vi "Search for User.vi"(0 "User Configuration Manager in":refnum<class "User Configuration Manager.lvclass">, 5 "Username":string, 11 "error in (no error)":errorcluster) -> (4 "User Configuration Manager out":refnum<class "User Configuration Manager.lvclass">, 6 "Found":bool, 15 "error out":errorcluster)   [LabVIEW 2017, in "User Configuration Manager.lvlib" / "User Configuration Manager.lvclass"]
uses:
  User Configuration Manager.lvclass
  User Configuration Manager.lvclass/User Configuration Manager.ctl
  Accessors/Read Linked List ID.vi
  Accessors/Read Linked List Ref .vi
  <vilib>/gpm_packages/@cs/linked-list/Source/Linked List/ILinkedList/ILinked List.lvclass
  <vilib>/gpm_packages/@cs/linked-list/Source/Linked List/Linked List Ref/Linked List Ref.lvclass
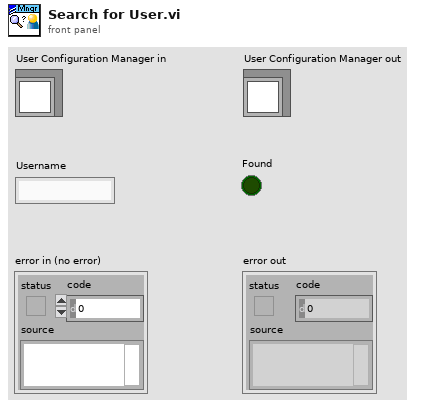
[diagram p1: front panel]
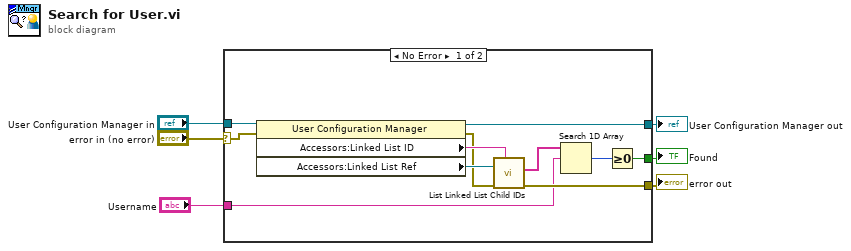
[diagram p0: block diagram]
diagram:
  n1 = case shown="No Error" "error in (no error)" {
    selector: "error in (no error)" -> [w11 w18]
    tunnel: "User Configuration Manager in" -> [w12 w19]
    tunnel: [w10 w19] -> w4
    tunnel: [w9 w18] -> w1
    tunnel: "Username" -> [w8 _]
    tunnel: [w7 _] -> w2
    frame No Error {
      n2 = property class="User Configuration Manager"(reference=w12, error in=w11) -> (reference out=w10:refnum<class "User Configuration Manager.lvclass">, error out=w14:errorcluster, "Accessors:Linked List ID"=w16:string, "Accessors:Linked List Ref "=w17:refnum<data-value>)
      n3 = call <vilib>:"List Linked List Child IDs.vi"("Linked List ID"=w16, "error in (no error)"=w14, "Linked List Ref"=w17) -> ("error out"=w9:errorcluster, "Child IDs"=w15:string[])  [unwired: 6 in, 1 out]
      n4 = Search 1D Array(1D array=w15, element=w8) -> (index of element=w13:i32)  [unwired: 1 in]
      n5 = Greater Or Equal To 0?(x=w13) -> (x >= 0?=w7:bool)
    }
    frame Error {
    }
  }
  "error out" <- w1
  "User Configuration Manager out" <- w4
  "Found" <- w2
